vi "Main - RT.vi"() -> ()   [LabVIEW 2020]
uses:
  Funktionstasten/Zustaende.ctl
  <vilib>/Platform/TimedLoop/XDataNode/timing_clust.ctl
  <vilib>/Platform/TimedLoop/XDataNode/nitl_modes.ctl
  <vilib>/Platform/TimedLoop/XDataNode/wakeup.ctl
  Konfig-Dateien/Aktionen Konfig.ctl
  Regler/Druckregler/Aktionen Interne Werte.ctl
  Allgemein/Aktion FGV Zustandsbeleuchtung schalten.ctl
  SysLog/SysLog Interface cRIO.ctl
  FGV Komm Status Aktionen.ctl
  <vilib>/Platform/TimedLoop/XDataNode/loadnilvce.vi
  <vilib>/Platform/TimedLoop/XDataNode/XDataNode.xnode
  <vilib>/Platform/TimedLoop/XDataNode/XDNodeRunTimeDep.lvlib
  Regler/Regler.lvlib
  Verwaltung/Verwaltung - cRIO.lvlib
  Kommunikation mit PC.lvlib
  Stoermeldungen/Stoermeldungen.lvlib
  Allgemein/Allgemein.lvlib
  Konfig-Dateien/Konfig-Dateien.lvlib
  Betriebsstundenzaehler/Betriebsstundenzaehler.lvlib
  Regler/Druckregler/Druckregler.lvlib
  Allgemein/Anlage Spuelen Aktionen.ctl
  SysLog/SysLog_cRIO.lvlib
  CAN Interface/CAN Interface.lvlib
  Funktionstasten/Funktionstasten.lvlib
panel:
  out "PID2":i32
  out "T PID 2":u32
  out "T BSZ":u32
  out "BSZ":i32
  out "Komm langsam":i32
  out "T Komm langsam":u32
  out "lebt PC?":bool
  out "T PID":u32
  out "T SPS":u32
  out "T Komm":u32
  out "T PWM":u32
  out "Zustand cRIO":T1
  out "PID":i32
  out "PWM":i32
  out "Komm":i32
  out "SPS":i32
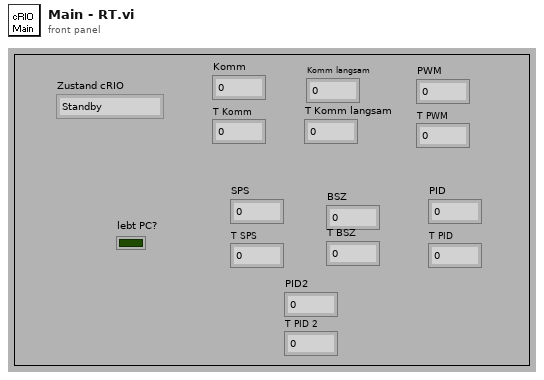
[diagram p1: front panel]
types:
  T1 = typedef "Funktionstasten.lvlib/Zustaende.ctl" = enum16{"Standby", "Pause", "Eco", "Messen", "Kalibrieren", "Spülen Filter", "Spülen Leitung", "Umgebungsluft", "0-Gas", "Cal-Gas", "CG zu PNS", "-------------", "Init 1", "Init 2", "Init 3", "Init 4", "Messen vorbereiten", "Messen durchführen", "Exit"}
  T2 = typedef "Allgemein.lvlib/Aktion FGV Zustandsbeleuchtung schalten.ctl" = enum16{"lesen", "prüfen", "init", "Bit löschen", "ansteuern", "Aufheizphase"}
  T3 = typedef "Konfig-Dateien.lvlib/Aktionen Konfig.ctl" = enum16{"lesen", "laden", "speichern  System.ini", "speichern Anlagengrenzw.", "speichern PID + Sonstige", "speichern BSZ BMP", "speichern BSZ FT-IR", "speichern Stickstoff Bef.", "speichern Ext. Stickstoff Bef.", "speichern CAN_Konfig"}
  T4 = typedef "Regler.lvlib/Druckregler.lvlib/Aktionen Interne Werte.ctl" = enum16{"lesen", "FT-IR", "Ausgang", "Pumpe", "laden", "speichern", "Änderung?", "Druck Kalter Block", "Dichtheitstest"}
  T5 = typedef "Allgemein.lvlib/Anlage Spuelen Aktionen.ctl" = enum16{"lesen", "spülen?"}
  T6 = typedef "SysLog_cRIO.lvlib/SysLog Interface cRIO.ctl" = cluster{"FehlermeldungsCode":i32, "ErfolgsmeldungsCode":i32, "ParameterListenString":string, "intern":bool}
  T7 = typedef "XDNodeRunTimeDep.lvlib/timing_clust.ctl" = cluster{"Expected End [f-1]":u64, "Actual End [f-1]":u64, "Finished Late? [f-1]":bool, "Expected End [i-1]":u64, "Actual End [i-1]":u64, "Finished Late? [i-1]":bool, "Expected Start [i]":u64, "Actual Start [i]":u64, "Expected Start [f]":u64, "Actual Start [f]":u64, "Source Name":string, "Structure Name":string, "Period":i64, "Deadline":i64, "Offset":i64, "Start":i64, "Priority":i32, "Timeout":i32, "Mode":T8, "Wakeup Reason":T9, "Error":errorcluster, "Source Type":string, "Secondary Source Type":string, "Global End Time":u64, "Global Start Time":u64, "Frame Duration":u64, "Iteration Duration":u64, "Assigned CPU":i32, "I/O Scan Engine Mode":u32}
  T8 = typedef "XDNodeRunTimeDep.lvlib/nitl_modes.ctl" = enum32{"No Change", "Process missed periods, maintain original phase", "Discard missed periods, maintain original phase", "Process missed periods, ignore original phase", "Discard missed periods, ignore original phase"}
  T9 = typedef "XDNodeRunTimeDep.lvlib/wakeup.ctl" = enum32{"Normal", "Aborted", "Asynchronous wakeup", "Timing source error", "Timed loop error", "Timeout"}
  T10 = typedef "Kommunikation mit PC.lvlib/FGV Komm Status Aktionen.ctl" = enum16{"lesen", "lebt PC?"}
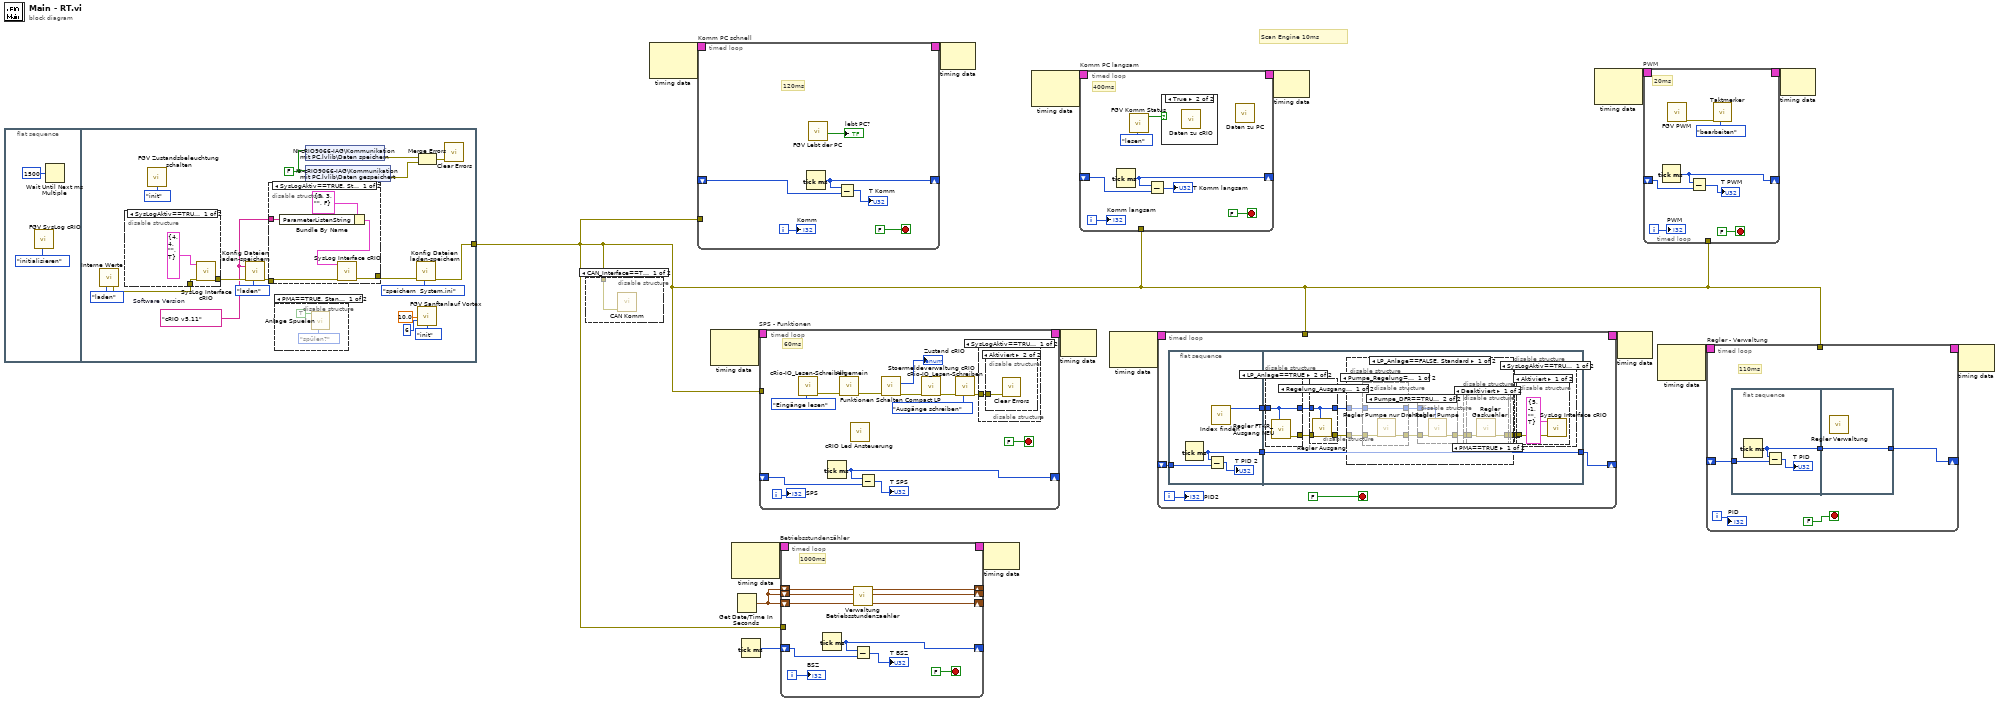
[diagram p0: block diagram]
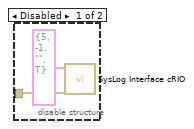
[diagram p3: hidden frame]
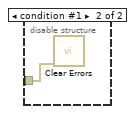
[diagram p4: hidden frame]
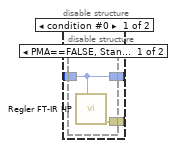
[diagram p6: hidden frame]
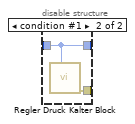
[diagram p7: hidden frame]
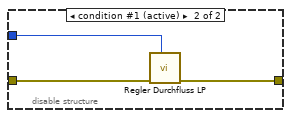
[diagram p12: hidden frame]
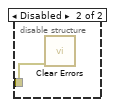
[diagram p13: hidden frame]
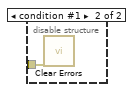
[diagram p14: hidden frame]
diagram:
  # "Scan Engine 10ms"
  n1 = flat-sequence {
    tunnel: [w36] -> w17
    frame #0 {
      n2 = call "FGV SysLog cRIO.vi"("Aktion"=enum16{"initialisieren", "lesen", "schreiben"}."initialisieren") -> ()  [unwired: 8 in, 3 out]
      n3 = Wait Until Next ms Multiple(millisecond multiple=u32 1500 ("ms")) -> ()  [unwired: 1 out]
    }
    frame #1 {
      w23 = "cRIO v5.11"  # Software Version
      w35 = FALSE ("Daten speichern")
      n4 = call "Interne Werte.vi"("Aktionen Interne Werte"=Aktionen_Interne_Werte."laden") -> ("error out"=w29:errorcluster)  [unwired: 8 in, 6 out]
      n5 = disable-structure shown="SysLogAktiv==TRUE" {
        disable-tunnel: w29 -> [w46 _]
        disable-tunnel: [w45 _] -> w28
        frame condition #0 (active) {
          n6 = call "SysLog Interface cRIO.vi"("Fehler (in)"=w46, "Cluster (in)"=T6 {"FehlermeldungsCode"=4, "ErfolgsmeldungsCode"=4, "ParameterListenString"="", "intern"=TRUE}) -> ("Fehler (Ausgang)"=w45:errorcluster)  [unwired: 9 in]
        }
        frame condition #1 {
        }
      }
      n7 = call "FGV Zustandsbeleuchtung schalten.vi"("Aktion"=Aktion_FGV_Zustandsbeleuchtung_schalten."init") -> ()  [unwired: 13 in, 2 out]
      n8 = call "Konfig Dateien laden-speichern.vi"("Aktion"=Aktionen_Konfig."laden", "Fehler (Eingang)"=w28, "Software Version"=w23) -> ("Fehler (Ausgang)"=w27:errorcluster)  [unwired: 8 in]
      n9 = disable-structure shown="SysLogAktiv==TRUE, Standard" {
        disable-tunnel: w27 -> [w43 _]
        disable-tunnel: [w42 _] -> w25
        disable-tunnel: w23 -> [w39 _]
        frame condition #0 (active) {
          n10 = Bundle By Name(cluster=T6 {"FehlermeldungsCode"=3, "ErfolgsmeldungsCode"=3, "ParameterListenString"="", "intern"=FALSE} ("Cluster (in)"), "ParameterListenString"=w39) -> (w40:T6)
          n11 = call "SysLog Interface cRIO.vi"("Fehler (in)"=w43, "Cluster (in)"=w40) -> ("Fehler (Ausgang)"=w42:errorcluster)  [unwired: 9 in]
        }
        frame condition #1 {
        }
      }
      n12 = disable-structure shown="PMA==TRUE, Standard" {
        frame condition #0 {
          n13 = call "Anlage Spuelen.vi"("Aktionen"=Anlage_Spuelen_Aktionen."spülen?", "Spülen?"=TRUE) -> ()  [unwired: 9 in, 1 out]
        }
        frame condition #1 (active) {
        }
      }
      n14 = shared-variable "NI-cRIO9066-IAG\\Kommunikation mit PC.lvlib\\Daten speichern"(w35) -> (error out=w31:errorcluster)  [unwired: 1 in]
      n15 = shared-variable "NI-cRIO9066-IAG\\Kommunikation mit PC.lvlib\\Daten gespeichert"(w35) -> (error out=w32:errorcluster)  [unwired: 1 in]
      n16 = call "Konfig Dateien laden-speichern.vi"("Aktion"=Aktionen_Konfig."speichern  System.ini", "Fehler (Eingang)"=w25) -> ("Fehler (Ausgang)"=w36:errorcluster)  [unwired: 9 in]
      n17 = call "FGV Sanftanlauf Vortex.vi"("Scantime Scanengine in ms"=10.0, "Perioden"=u32 6, "Aktion"=enum16{"init", "aktiv"}."init") -> ()  [unwired: 11 in, 2 out]
      n18 = Merge Errors(w31, w32) -> (w30:errorcluster)
      n19 = call <vilib>:"Clear Errors.vi"("error in (no error)"=w30) -> ()  [unwired: 5 in, 2 out]
    }
  }
  n20 = disable-structure shown="CAN_Interface==TRUE, Standard" {
    disable-tunnel: w17 -> [w47 _]
    frame condition #0 {
      n21 = call "CAN Komm.vi"("error in"=w47) -> ()  [unwired: 10 in, 1 out]
    }
    frame condition #1 (active) {
    }
  }
  n22 = node-c288() -> (w16:T7)  [unwired: 2 out]
  n23 = timed-loop "Komm PC schnell" {
    timing: w16 -> [_]
    timing-out: [_] -> w15
    shift-right: [w50] -> _
    shift-left: _ -> [w51]
    tunnel: w17 -> [_]
    i -> [w52]
    stop <- FALSE stop-if-true
    # "120ms"
    n24 = Tick Count (ms)() -> (millisecond timer value=w50:u32)
    n25 = call "FGV Lebt der PC.vi"() -> ("lebt PC?"=→"lebt PC?":bool)  [unwired: 11 in]
    n26 = Subtract(x=w50, y=w51) -> (x-y=→"T Komm":u32)
    "Komm" <- w52
  }
  n27 = node-c288() -> (w2:T7)  [unwired: 2 out]
  n28 = node-c288() -> (w6:T7)  [unwired: 2 in]
  n29 = Get Date/Time In Seconds() -> (seconds since 1Jan1904=w3:timestamp)
  n30 = Tick Count (ms)() -> (millisecond timer value=w4:u32)
  n31 = timed-loop "SPS - Funktionen" {
    timing: w2 -> [_]
    timing-out: [_] -> w1
    shift-right: [w57] -> _
    shift-left: _ -> [w58]
    tunnel: w17 -> [_]
    i -> [w67]
    stop <- FALSE stop-if-true
    # "60ms"
    n32 = call "cRio-IO_Lesen-Schreiben.vi"("Aktion"=enum16{"Eingänge lesen", "Ausgänge schreiben"}."Eingänge lesen") -> ("Fehler Ausgang"=w64:errorcluster)  [unwired: 10 in]
    n33 = Tick Count (ms)() -> (millisecond timer value=w57:u32)
    n34 = call "Allgemein.vi"("Fehler (Eingang)"=w64) -> ("Fehler (Ausgang)"=w63:errorcluster)  [unwired: 10 in]
    n35 = call "cRIO Led Ansteuerung.vi"() -> ()  [unwired: 11 in, 1 out]
    n36 = Subtract(x=w57, y=w58) -> (x-y=→"T SPS":u32)
    n37 = call "Funktionen Schalten Compact LP.vi"("Fehler (Eingang)"=w63) -> ("Fehler (Ausgang)"=w65:errorcluster, "Zustand"=→"Zustand cRIO":T1)  [unwired: 9 in]
    n38 = call "Stoermeldeverwaltung cRIO.vi"("Fehler (Eingang)"=w65) -> ("Fehler (Ausgang)"=w60:errorcluster)  [unwired: 10 in]
    n39 = call "cRio-IO_Lesen-Schreiben.vi"("Aktion"=enum16{"Eingänge lesen", "Ausgänge schreiben"}."Ausgänge schreiben", "Fehler Eingang"=w60) -> ("Fehler Ausgang"=w56:errorcluster)  [unwired: 9 in]
    n40 = disable-structure shown="SysLogAktiv==TRUE" {
      disable-tunnel: w56 -> [w69 w73]
      frame condition #0 (active) {
        n41 = disable-structure shown="Aktiviert" {
          disable-tunnel: w69 -> [w71 w72]
          frame Disabled {
            n42 = call "SysLog Interface cRIO.vi"("Fehler (in)"=w71, "Cluster (in)"=T6 {"FehlermeldungsCode"=5, "ErfolgsmeldungsCode"=-1, "ParameterListenString"="", "intern"=TRUE}) -> ()  [unwired: 9 in, 1 out]
          }
          frame Enabled {
            n43 = call <vilib>:"Clear Errors.vi"("error in (no error)"=w72) -> ()  [unwired: 5 in, 2 out]
          }
        }
      }
      frame condition #1 {
        n44 = call <vilib>:"Clear Errors.vi"("error in (no error)"=w73) -> ()  [unwired: 5 in, 2 out]
      }
    }
    "SPS" <- w67
  }
  n45 = timed-loop "Betriebsstundenzähler" {
    timing: w6 -> [_]
    timing-out: [_] -> w5
    shift-right: [w83] -> _
    shift-left: w4 -> [w84]
    shift-right: [w79] -> _
    shift-left: w3 -> [w81]
    shift-right: [w78] -> _
    shift-left: w3 -> [w80]
    tunnel: w17 -> [_]
    shift-right: [w77] -> _
    shift-left: w3 -> [w76]
    i -> [w85]
    stop <- FALSE stop-if-true
    # "1000ms"
    n46 = Tick Count (ms)() -> (millisecond timer value=w83:u32)
    n47 = call "Verwaltung Betriebsstundenzaehler.vi"("Zeitstempel Syslog"=w80, "Zeitstempel FT-IR"=w76, "Zeitstempel BMP"=w81) -> ("Zeitstempel Syslog"=w78:timestamp, "Zeitstempel FT-IR"=w77:timestamp, "Zeitstempel BMP"=w79:timestamp)  [unwired: 6 in]
    n48 = Subtract(x=w83, y=w84) -> (x-y=→"T BSZ":u32)
    "BSZ" <- w85
  }
  n49 = node-c288(w15) -> ()  [unwired: 1 out]
  n50 = node-c288(w5) -> ()  [unwired: 1 out]
  n51 = node-c288() -> (w14:T7)  [unwired: 2 in]
  n52 = node-c288(w1) -> ()  [unwired: 1 out]
  n53 = timed-loop "Komm PC langsam" {
    timing: w14 -> [_]
    timing-out: [_] -> w13
    shift-right: [w93] -> _
    shift-left: _ -> [w94]
    tunnel: w17 -> [_]
    i -> [w91]
    stop <- FALSE stop-if-true
    # "400ms"
    n54 = Tick Count (ms)() -> (millisecond timer value=w93:u32)
    n55 = call "FGV Komm Status.vi"("Aktionen"=FGV_Komm_Status_Aktionen."lesen") -> ("lebt PC?"=w89:bool)  [unwired: 10 in]
    n56 = Subtract(x=w93, y=w94) -> (x-y=→"T Komm langsam":u32)
    n57 = case shown="True" w89 {
      frame False {
      }
      frame True {
        n58 = call "Daten zu cRIO.vi"() -> ()  [unwired: 1 out]
      }
    }
    n59 = call "Daten zu PC.vi"() -> ()  [unwired: 1 out]
    "Komm langsam" <- w91
  }
  n60 = node-c288() -> (w12:T7)  [unwired: 2 in]
  n61 = timed-loop {
    timing: w12 -> [_]
    timing-out: [_] -> w11
    shift-right: [w100] -> _
    shift-left: _ -> [w101]
    tunnel: w17 -> [_]
    i -> [w99]
    stop <- FALSE stop-if-true
    n62 = flat-sequence {
      tunnel: w101 -> [w106]
      tunnel: [w105] -> w102
      tunnel: [w104] -> w98
      tunnel: [w114] -> w100
      tunnel: w102 -> [w114]
      tunnel: w98 -> [w110]
      frame #0 {
        n63 = Tick Count (ms)() -> (millisecond timer value=w105:u32)
        n64 = Subtract(x=w105, y=w106) -> (x-y=→"T PID 2":u32)
        n65 = call "Index finden.vi"() -> ("Index"=w104:i32)  [unwired: 11 in]
      }
      frame #1 {
        n66 = disable-structure shown="LP_Anlage==TRUE" {
          disable-tunnel: [w122 w127] -> w112
          disable-tunnel: w110 -> [w121 w128]
          disable-tunnel: [w120 w128] -> w109
          frame condition #0 {
            n67 = disable-structure shown="PMA==FALSE, Standard" {
              disable-tunnel: [w124 w126] -> w122
              disable-tunnel: w121 -> [w123 w125]
              disable-tunnel: [w123 w125] -> w120
              frame condition #0 (active) {
                n68 = call "Regler FT-IR HP.vi"("Index"=w123) -> ("Fehler (Ausgang)"=w124:errorcluster)  [unwired: 10 in]
              }
              frame condition #1 {
                n69 = call "Regler Druck Kalter Block.vi"("Index"=w125) -> ("Fehler (Ausgang)"=w126:errorcluster)  [unwired: 10 in]
              }
            }
          }
          frame condition #1 (active) {
            n70 = call "Regler FT-IR_Ausgang NEU.vi"("Index"=w128) -> ("Fehler (Ausgang)"=w127:errorcluster)  [unwired: 10 in]
          }
        }
        n71 = disable-structure shown="Regelung_Ausgang_vorhanden==TRUE, Standard" {
          disable-tunnel: [w117 w118] -> w113
          disable-tunnel: w112 -> [w116 w118]
          disable-tunnel: w109 -> [w115 w119]
          disable-tunnel: [w115 w119] -> w108
          frame condition #0 (active) {
            n72 = call "Regler Ausgang.vi"("Index"=w115, "Fehler"=w116) -> ("Fehler (Ausgang)"=w117:errorcluster)  [unwired: 9 in]
          }
          frame condition #1 {
          }
        }
        n73 = disable-structure shown="LP_Anlage==FALSE, Standard" {
          disable-tunnel: w113 -> [w134 w152]
          disable-tunnel: [w133 w151] -> w111
          disable-tunnel: w108 -> [w132 w150]
          frame condition #0 {
            n74 = disable-structure shown="Pumpe_Regelung==TRUE" {
              disable-tunnel: w134 -> [w147 w149]
              disable-tunnel: [w146 w149] -> w131
              disable-tunnel: w132 -> [w145 w148]
              disable-tunnel: [w145 w148] -> w129
              frame condition #0 {
                n75 = call "Regler Pumpe nur Drehzahl.vi"("Fehler"=w147) -> ("Fehler (Ausgang)"=w146:errorcluster)  [unwired: 10 in]
              }
              frame condition #1 (active) {
              }
            }
            n76 = disable-structure shown="Pumpe_DFR==TRUE, Standard" {
              disable-tunnel: w131 -> [w141 w144]
              disable-tunnel: [w141 w143] -> w130
              disable-tunnel: w129 -> [_ w142]
              frame condition #0 {
              }
              frame condition #1 (active) {
                n77 = call "Regler Pumpe.vi"("Index"=w142, "Fehler"=w144) -> ("Fehler (Ausgang)"=w143:errorcluster)  [unwired: 9 in]
              }
            }
            n78 = disable-structure shown="Deaktiviert" {
              disable-tunnel: [w136 w140] -> w133
              disable-tunnel: w130 -> [w135 w140]
              frame Disabled {
                n79 = disable-structure shown="PMA==TRUE" {
                  disable-tunnel: w135 -> [w138 w139]
                  disable-tunnel: [w137 w139] -> w136
                  frame condition #0 {
                    n80 = call "Regler Gaskuehler.vi"("Fehler"=w138) -> ("Fehler (Ausgang)"=w137:errorcluster)  [unwired: 10 in]
                  }
                  frame condition #1 (active) {
                  }
                }
              }
              frame Enabled {
              }
            }
          }
          frame condition #1 (active) {
            n81 = call "Regler Durchfluss LP.vi"("Index"=w150, "Fehler"=w152) -> ("Fehler (Ausgang)"=w151:errorcluster)  [unwired: 9 in]
          }
        }
        n82 = disable-structure shown="SysLogAktiv==TRUE" {
          disable-tunnel: w111 -> [w153 w157]
          frame condition #0 (active) {
            n83 = disable-structure shown="Aktiviert" {
              disable-tunnel: w153 -> [w155 w156]
              frame Enabled {
                n84 = call "SysLog Interface cRIO.vi"("Fehler (in)"=w155, "Cluster (in)"=T6 {"FehlermeldungsCode"=5, "ErfolgsmeldungsCode"=-1, "ParameterListenString"="", "intern"=TRUE}) -> ()  [unwired: 9 in, 1 out]
              }
              frame Disabled {
                n85 = call <vilib>:"Clear Errors.vi"("error in (no error)"=w156) -> ()  [unwired: 5 in, 2 out]
              }
            }
          }
          frame condition #1 {
            n86 = call <vilib>:"Clear Errors.vi"("error in (no error)"=w157) -> ()  [unwired: 5 in, 2 out]
          }
        }
      }
    }
    "PID2" <- w99
  }
  n87 = node-c288(w13) -> ()  [unwired: 1 out]
  n88 = node-c288() -> (w10:T7)  [unwired: 2 out]
  n89 = node-c288(w11) -> ()  [unwired: 1 out]
  n90 = timed-loop "PWM" {
    timing: w10 -> [_]
    timing-out: [_] -> w9
    shift-right: [w161] -> _
    shift-left: _ -> [w160]
    tunnel: w17 -> [_]
    i -> [w165]
    stop <- FALSE stop-if-true
    # "20ms"
    n91 = Tick Count (ms)() -> (millisecond timer value=w161:u32)
    n92 = call "FGV PWM.vi"() -> ("error out"=w163:errorcluster)  [unwired: 11 in]
    n93 = Subtract(x=w161, y=w160) -> (x-y=→"T PWM":u32)
    n94 = call "Taktmerker.vi"("Aktion"=enum16{"lesen", "bearbeiten"}."bearbeiten", "error in"=w163) -> ()  [unwired: 5 in, 5 out]
    "PWM" <- w165
  }
  n95 = node-c288() -> (w8:T7)  [unwired: 2 out]
  n96 = timed-loop "Regler - Verwaltung" {
    timing: w8 -> [_]
    timing-out: [_] -> w7
    shift-right: [w170] -> _
    shift-left: _ -> [w171]
    tunnel: w17 -> [_]
    i -> [w172]
    stop <- FALSE stop-if-true
    # "110ms"
    n97 = flat-sequence {
      tunnel: w171 -> [w175]
      tunnel: [w174] -> w169
      tunnel: [w177] -> w170
      tunnel: w169 -> [w177]
      frame #0 {
        n98 = Tick Count (ms)() -> (millisecond timer value=w174:u32)
        n99 = Subtract(x=w174, y=w175) -> (x-y=→"T PID":u32)
      }
      frame #1 {
        n100 = call "Regler Verwaltung.vi"() -> ()  [unwired: 11 in, 1 out]
      }
    }
    "PID" <- w172
  }
  n101 = node-c288(w9) -> ()  [unwired: 1 out]
  n102 = node-c288(w7) -> ()  [unwired: 1 out]
